vi "Test Strict Find Items as LV Type2.vi"(11 "Test Case In":refnum<class "Test Strict Find Items as LV Type.lvclass">) -> (0 "error out":errorcluster, 3 "Test Case Out":refnum<class "Test Strict Find Items as LV Type.lvclass">)   [LabVIEW 2023, in "Test Strict Find Items as LV Type.lvclass"]
uses:
  Test Strict Find Items as LV Type.lvclass
  C:/Program Files/National Instruments/LabVIEW 2023/vi.lib/Astemes/LUnit/Test Case.lvclass
  <vilib>/Astemes/LUnit/Test Case.lvclass/Test Case.ctl
  3569c10e-a7e7-4a2f-bada-2f7c60693600.vi
  3569c10e-a7e7-4a2f-bada-2f7c60693600.vi/a4169a97-72fc-4003-a778-603cf20cafa0.vi
  <vilib>/Astemes/LUnit/Append Fail Result.vi
  <vilib>/Astemes/LUnit/Append Pass Result.vi
  <vilib>/JDP Science/JSONtext/Find Item.vi
  <vilib>/Astemes/LUnit/Run In UI.vi
  <vilib>/JDP Science/JSONtext/Next JSON Value.vi
  <vilib>/JDP Science/JSONtext/String Subset.vi
  <vilib>/Utility/error.llb/Clear Errors.vi
  <vilib>/JDP Science/JSONtext/Parsing/Advance past next JSON Value (inlined COPY).vi
  <vilib>/JDP Science/JSONtext/Parsing/Advance past whitespace.vi
  <vilib>/JDP Science/JSONtext/Parsing/Advance past String.vi
  <vilib>/JDP Science/JSONtext/Parsing/Advance past Number.vi
  <vilib>/JDP Science/JSONtext/Parsing/Advance past Line Ending.vi
  <vilib>/JDP Science/JSONtext/Parsing/Parse Full Path or Item Name.vi
  <vilib>/JDP Science/JSONtext/Parsing/Advance past Array.vi
  <vilib>/JDP Science/JSONtext/Parsing/Advance past Object.vi
  <vilib>/JDP Science/JSONtext/support/Error Cluster From Code.vi
  <vilib>/JDP Science/JSONtext/Offset/Find Item Locations by Path.vi
  <vilib>/JDP Science/JSONtext/JSON text to Variant.vi
  <vilib>/Utility/error.llb/Error Cluster From Error Code.vi
  <vilib>/JDP Science/JSONtext/LVClass Serializer/JSONtext LVClass Serializer.lvclass
  <vilib>/Astemes/LUnit/Test Case.lvclass
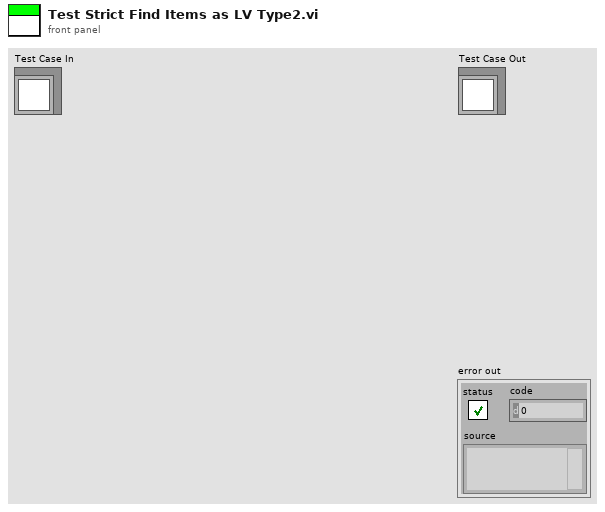
[diagram p1: front panel]
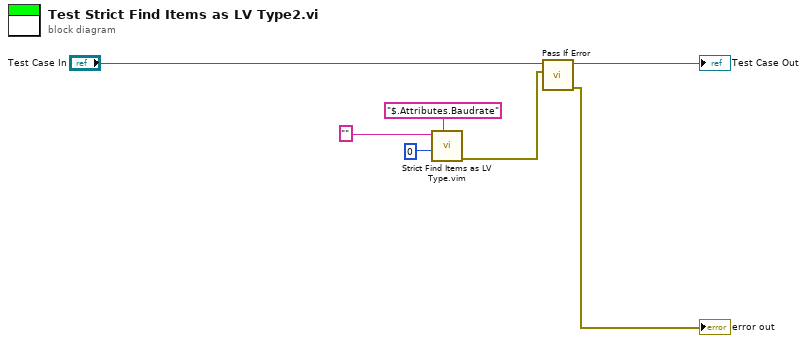
[diagram p0: block diagram]
diagram:
  n1 = call "Strict Find Items as LV Type.vim"("$Path or Item Name"="$.Attributes.Baudrate", "Data Type and Default Value"=u16 0, "JSON"="") -> ("error out"=w1:errorcluster)  [unwired: 7 in, 1 out]
  n2 = call <vilib>:"Pass If Error.vi"("Assert error"=w1, "LUnit Test Case In"="Test Case In") -> ("error out"=→"error out":errorcluster, "LUnit Test Case Out"=→"Test Case Out":refnum<class "Test Strict Find Items as LV Type.lvclass">)  [unwired: 8 in]
